vi "draw_plot.vi"(8 "error in (no error)":errorcluster, 10 "Dataset":T1(array[cluster]), 11 "handle":i32) -> (0 "error out":errorcluster, 3 "Plot":cluster{dbl[], dbl[]})   [LabVIEW 2018]
uses:
  <userlib>/Gigahertz-Optik/GOMDTR9600/GOMDTR9600.lvlib
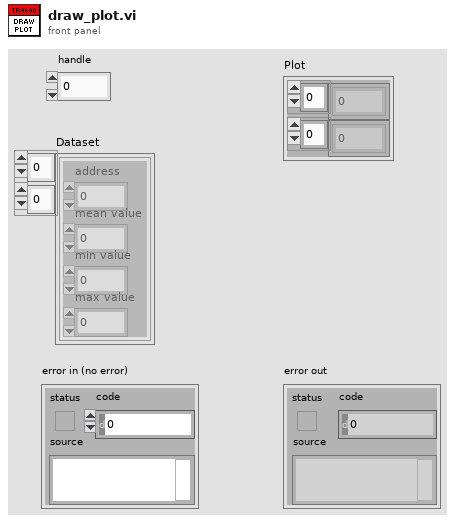
[diagram p1: front panel]
types:
  T1 = cluster{"address":i32, "mean value":dbl, "min value":dbl, "max value":dbl}[][]
  T2 = cluster{"address":i32, "mean value":dbl, "min value":dbl, "max value":dbl}[]
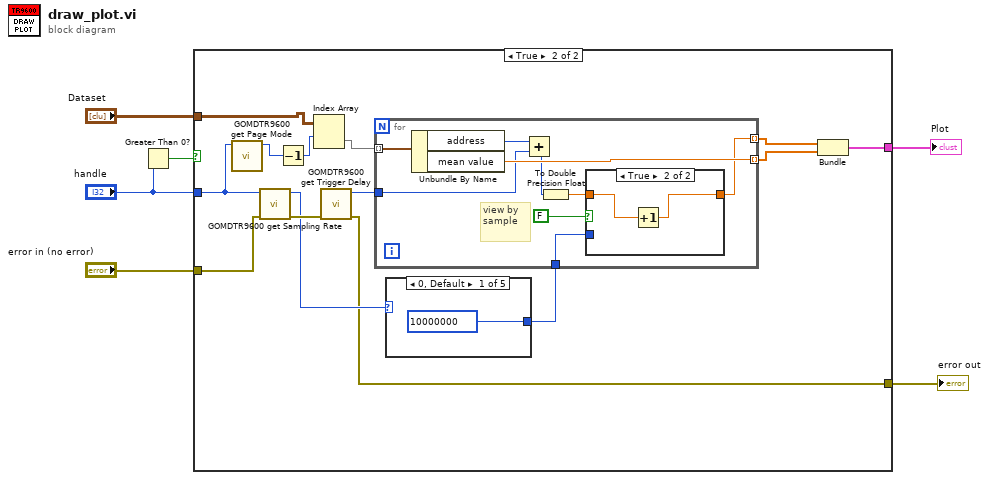
[diagram p0: block diagram]
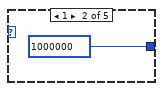
[diagram p3: hidden frame]
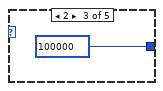
[diagram p4: hidden frame]
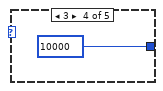
[diagram p5: hidden frame]
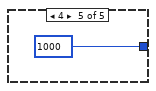
[diagram p6: hidden frame]
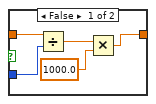
[diagram p7: hidden frame]
diagram:
  n1 = Greater Than 0?(x="handle") -> (x > 0?=w1:bool)
  n2 = case shown="True" w1 {
    tunnel: [_ w19] -> w6
    tunnel: "Dataset" -> [_ w11]
    tunnel: "error in (no error)" -> [w7 w14]
    tunnel: "handle" -> [_ w12]
    tunnel: [w7 w13] -> w3
    frame False {
    }
    frame True {
      n3 = call <userlib>:"GOMDTR9600 get Page Mode.vi"("handle"=w12) -> ("value"=w9:i32)  [unwired: 8 in, 2 out]
      n4 = call <userlib>:"GOMDTR9600 get Sampling Rate.vi"("error in (no error)"=w14, "handle"=w12) -> ("error out"=w20:errorcluster, "value"=w16:i32)  [unwired: 7 in, 1 out]
      n5 = Decrement(x=w9) -> (x-1=w8:i32)
      n6 = Index Array(array=w11, index (row)=w8) -> (element=w10:T2)  [unwired: 1 in]
      n7 = call <userlib>:"GOMDTR9600 get Trigger Delay.vi"("error in (no error)"=w20) -> ("error out"=w13:errorcluster, "value"=w15:i32)  [unwired: 8 in, 1 out]
      n8 = case shown="0, Default" w16 {
        tunnel: [10000000 ("value") 1000000 ("value") 100000 ("value") 10000 ("value") 1000 ("value")] -> w21
        frame 0, Default {
        }
        frame 1 {
        }
        frame 2 {
        }
        frame 3 {
        }
        frame 4 {
        }
      }
      n9 = for {
        tunnel: w10 -> [w35] mode=indexing
        tunnel: [w34] -> w18 mode=indexing
        tunnel: [w32] -> w17 mode=indexing
        tunnel: w15 -> [w31]
        tunnel: w21 -> [w27]
        # "view by\nsample"
        n10 = Unbundle By Name(w35) -> ("address"=w30:i32, "mean value"=w34:dbl)
        n11 = Add(x=w30, y=w31) -> (x+y=w29:i32)
        n12 = To Double Precision Float(number=w29) -> (double precision float=w33:dbl)
        n13 = case shown="True" FALSE {
          tunnel: w33 -> [w40 w42]
          tunnel: [w37 w41] -> w32
          tunnel: w27 -> [w36 _]
          frame False {
            n14 = Divide(x=w40, y=w36) -> (x/y=w39:dbl)
            n15 = Multiply(x=w39, y=1000.0) -> (x*y=w37:dbl)
          }
          frame True {
            n16 = Increment(x=w42) -> (x+1=w41:dbl)
          }
        }
      }
      n17 = Bundle(w17, w18) -> (w19:cluster{dbl[], dbl[]})  [unwired: 1 in]
    }
  }
  "Plot" <- w6
  "error out" <- w3
